vi "Simulation Kobuki Drive.vi"(8 "error in":errorcluster, 10 "sensors":T2 {"accelerometer"."z axis (g)" format="%.3f"; "accelerometer"."y axis (g)" format="%.3f"; "accelerometer"."x axis (g)" format="%.3f"}, 11 "Robot In":T1) -> (0 "error out":errorcluster, 2 "sensors":T2 {"accelerometer"."z axis (g)" format="%.3f"; "accelerometer"."y axis (g)" format="%.3f"; "accelerometer"."x axis (g)" format="%.3f"}, 3 "Robot Out":T1)   [LabVIEW 2014]
uses:
  shared/Sensors.ctl
  shared/Accelerometer.ctl
  Kobuki/KobukiSensors.ctl
  Kobuki/Kobuki Bumps and WheelDrops.ctl
  Kobuki/Kobuki Buttons.ctl
  Kobuki/Charging Sources Available.ctl
  Multi Bot Code/RobotData.ctl
  <instrlib>/DC Motor Controller/HAIOL/DC Motor Controller.lvclass
panel:
  # "Electrical: charging, battery, OI mode"
  # "Sensors: bump, cliff, button, wheel drop, wall, virtual wall"
  # "Motors:"
  # "Song"
  # "Inertia"
  # "Electrical: charging, battery, OI mode"
  # "Sensors: bump, cliff, button, wheel drop, wall, virtual wall"
  # "Motors:"
  # "Song"
  # "Inertia"
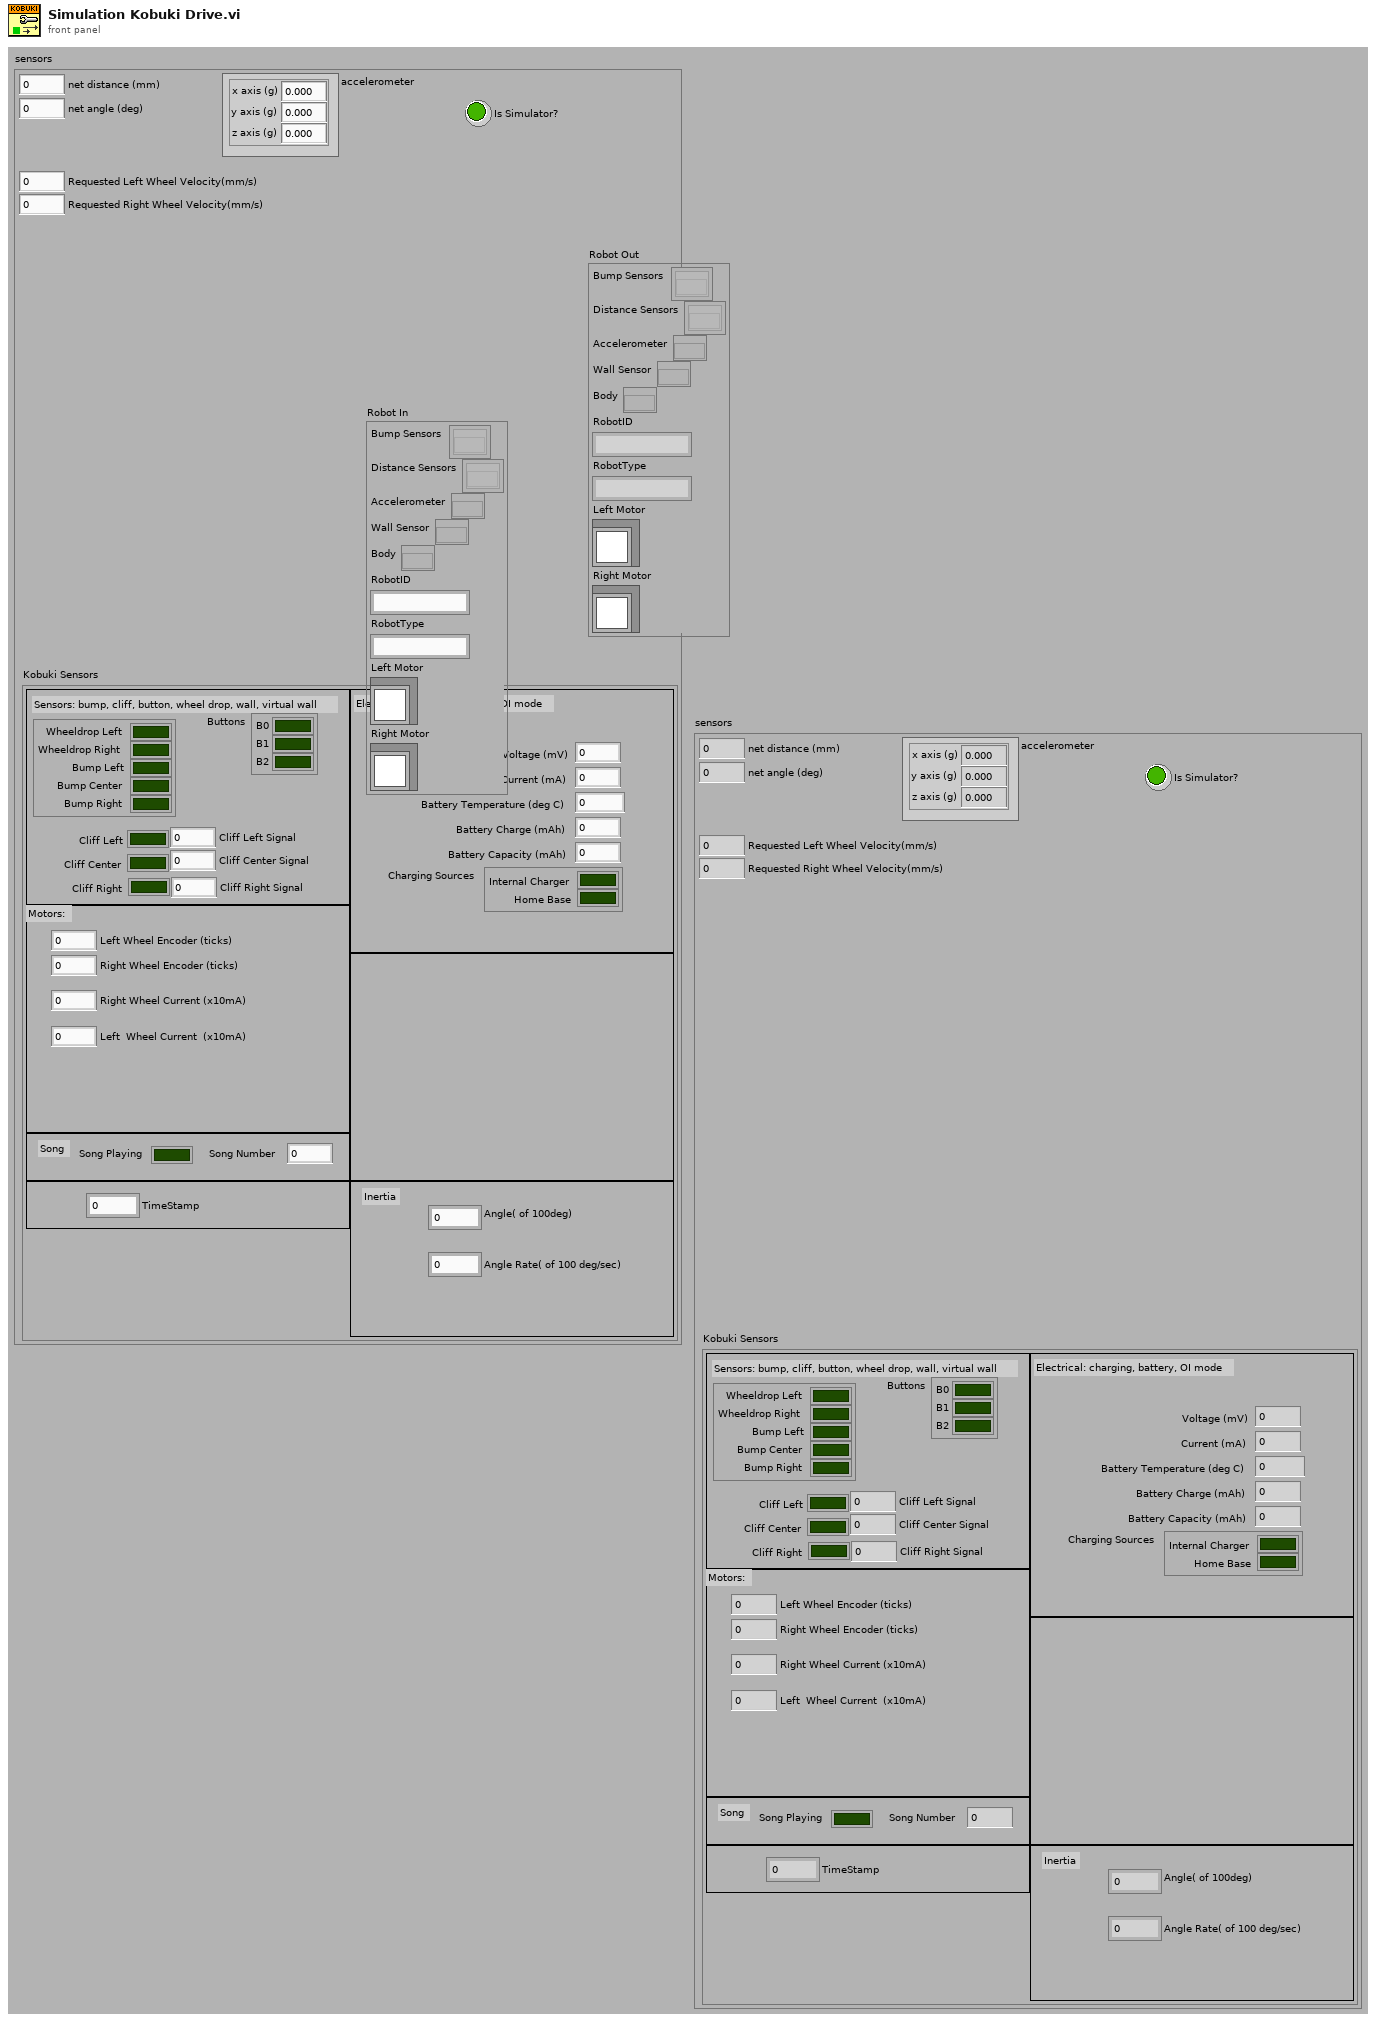
[diagram p1: front panel]
types:
  T1 = typedef "RobotData.ctl" = cluster{"Bump Sensors":refnum<k20>[], "Distance Sensors":refnum<k20>[], "Accelerometer":refnum<k20>, "Wall Sensor":refnum<k20>, "Body":refnum<k20>, "RobotID":string, "RobotType":string, "Left Motor":refnum<class "DC Motor Controller.lvclass">, "Right Motor":refnum<class "DC Motor Controller.lvclass">}
  T2 = typedef "Sensors.ctl" = cluster{"net distance (mm)":i32, "net angle (deg)":i32, "accelerometer":T3, "Is Simulator?":bool, "Kobuki Sensors":T4, "Requested Left Wheel Velocity(mm/s)":i32, "Requested Right Wheel Velocity(mm/s)":i32}
  T3 = typedef "Accelerometer.ctl" = cluster{"x axis (g)":dbl, "y axis (g)":dbl, "z axis (g)":dbl}
  T4 = typedef "KobukiSensors.ctl" = cluster{"Bumps + Wheel Drops":T5, "Cliff Left":bool, "Cliff Center":bool, "Cliff Right":bool, "Cliff Left Signal":u16, "Cliff Center Signal":u16, "Cliff Right Signal":u16, "Buttons":T6, "Left Wheel Encoder (ticks)":u16, "Right Wheel Encoder (ticks) ":u16, "Right Wheel Current (x10mA)":i16, "Left  Wheel Current  (x10mA)":i16, "TimeStamp":u16, "Song Playing":bool, "Song Number":u8, "Voltage (mV)":i16, "Current (mA)":i16, "Battery Temperature (deg C)":i16, "Battery Charge (mAh)":i16, "Battery Capacity (mAh)":i16, "Charging Sources":T7, "Angle( of 100deg)":i16, "Angle Rate( of 100 deg/sec)":i16}
  T5 = typedef "Kobuki Bumps and WheelDrops.ctl" = cluster{"Wheeldrop Left":bool, "Wheeldrop Right":bool, "Bump Left":bool, "Bump Center":bool, "Bump Right":bool}
  T6 = typedef "Kobuki Buttons.ctl" = cluster{"B0":bool, "B1":bool, "B2":bool}
  T7 = typedef "Charging Sources Available.ctl" = cluster{"Internal Charger":bool, "Home Base":bool}
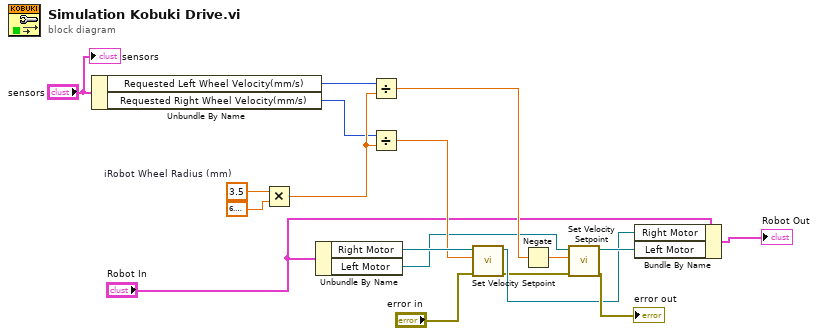
[diagram p0: block diagram]
diagram:
  w17 = 3.5  # iRobot Wheel Radius (mm)
  n1 = Unbundle By Name("sensors") -> ("Requested Left Wheel Velocity(mm/s)"=w4:i32, "Requested Right Wheel Velocity(mm/s)"=w3:i32)
  n2 = Multiply(x=w17, y=6.283185307179586) -> (x*y=w15:dbl)
  n3 = Unbundle By Name("Robot In") -> ("Right Motor"=w14:refnum<class "DC Motor Controller.lvclass">, "Left Motor"=w11:refnum<class "DC Motor Controller.lvclass">)
  n4 = Divide(x=w4, y=w15) -> (x/y=w18:dbl)
  n5 = Divide(x=w3, y=w15) -> (x/y=w13:dbl)
  n6 = call-dynamic "Set Velocity Setpoint.vi"("error in (no error)"="error in", "CCW Velocity (0 rad/s)"=w13, "DC Motor Controller in"=w14) -> ("error out"=w6:errorcluster, "DC Motor Controller out"=w7:refnum<class "DC Motor Controller.lvclass">)  [unwired: 7 in]
  n7 = Negate(x=w18) -> (-x=w10:dbl)
  n8 = call-dynamic "Set Velocity Setpoint.vi"("error in (no error)"=w6, "CCW Velocity (0 rad/s)"=w10, "DC Motor Controller in"=w11) -> ("error out"=→"error out":errorcluster, "DC Motor Controller out"=w8:refnum<class "DC Motor Controller.lvclass">)  [unwired: 7 in]
  n9 = Bundle By Name(cluster="Robot In", "Right Motor"=w7, "Left Motor"=w8) -> (→"Robot Out":T1)
  "sensors" <- "sensors"
